vi "car_spec.vi"(11 "Car_name":string) -> (0 "turn radius":dbl=5.50164, 1 "wheel base":dbl=25.77230806 format="%#_12g", 2 "ratio":dbl=25.77230806 format="%#_12g", 3 "overall width":dbl=1.77546, 4 "maximum steering angle [deg]":dbl, 5 "af":dbl)   [LabVIEW 2015]
panel:
  out "Car_name out":string
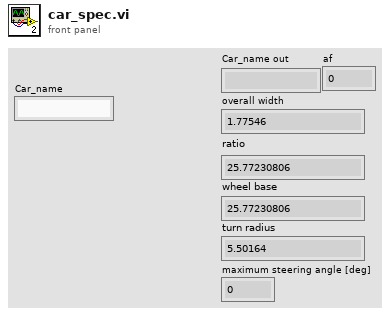
[diagram p1: front panel]
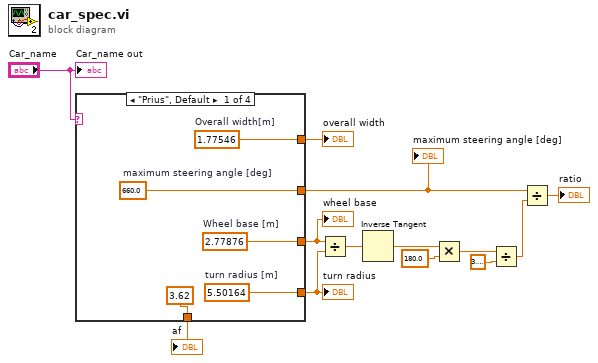
[diagram p0: block diagram]
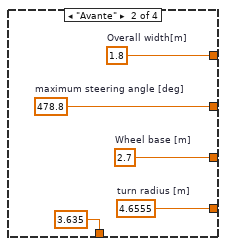
[diagram p2: hidden frame]
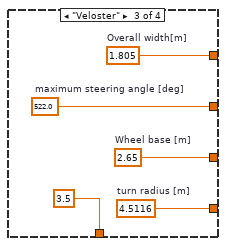
[diagram p3: hidden frame]
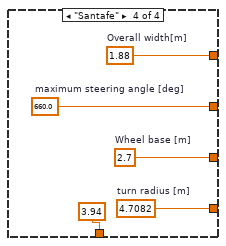
[diagram p4: hidden frame]
diagram:
  n1 = case shown="\"Prius\", Default" "Car_name" {
    tunnel: [w18 w23 w28 w33] -> w13
    tunnel: [w17 w22 w27 w32] -> w3
    tunnel: [w16 w21 w26 w31] -> w5
    tunnel: [w15 w20 w25 w30] -> w2
    tunnel: [3.62 3.635 3.5 3.94] -> w1
    frame "Prius", Default {
      w16 = 1.77546  # Overall width[m]
      w18 = 660.0  # maximum steering angle [deg]
      w15 = 5.50164  # turn radius [m]
      w17 = 2.77876  # Wheel base [m]
    }
    frame "Avante" {
      w21 = 1.8  # Overall width[m]
      w23 = 478.8  # maximum steering angle [deg]
      w20 = 4.6555  # turn radius [m]
      w22 = 2.7  # Wheel base [m]
    }
    frame "Veloster" {
      w26 = 1.805  # Overall width[m]
      w28 = 522.0  # maximum steering angle [deg]
      w25 = 4.5116  # turn radius [m]
      w27 = 2.65  # Wheel base [m]
    }
    frame "Santafe" {
      w31 = 1.88  # Overall width[m]
      w33 = 660.0  # maximum steering angle [deg]
      w30 = 4.7082  # turn radius [m]
      w32 = 2.7  # Wheel base [m]
    }
  }
  "overall width" <- w5
  "wheel base" <- w3
  "turn radius" <- w2
  "maximum steering angle [deg]" <- w13
  "af" <- w1
  n2 = Divide(x=w3, y=w2) -> (x/y=w7:dbl)
  n3 = Inverse Tangent(1:w7) -> (0:w11:dbl)
  n4 = Multiply(x=w11, y=180.0) -> (x*y=w9:dbl)
  n5 = Divide(x=w9, y=3.141592653589793) -> (x/y=w12:dbl)
  n6 = Divide(x=w13, y=w12) -> (x/y=→"ratio":dbl)
  "Car_name out" <- "Car_name"
